vi "sendMessage.vi"(8 "error in (no error)":errorcluster, 10 "message":string, 11 "SpectrographClientCommunicator in":refnum<class "SpectrographClientCommunicator.lvclass">) -> (0 "error out":errorcluster, 3 "SpectrographClientCommunicator out":refnum<class "SpectrographClientCommunicator.lvclass">)   [LabVIEW 2016, in "SpectrographClientCommunicator.lvclass"]
uses:
  SpectrographClientCommunicator.lvclass
  ts_labview_tcp/TCPClient/TCPClient.lvclass
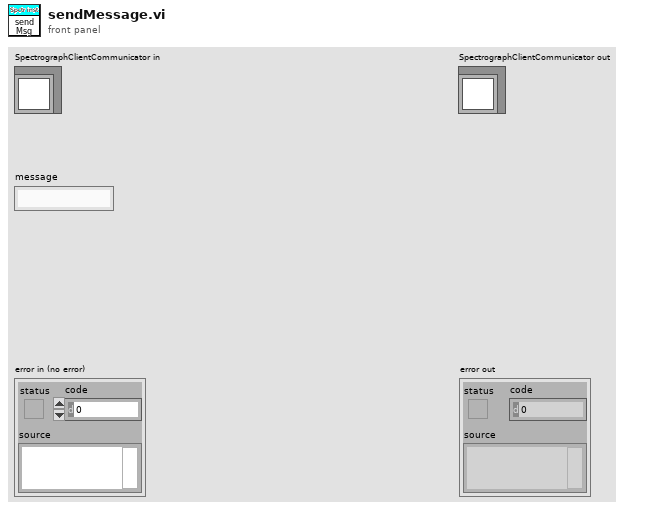
[diagram p1: front panel]
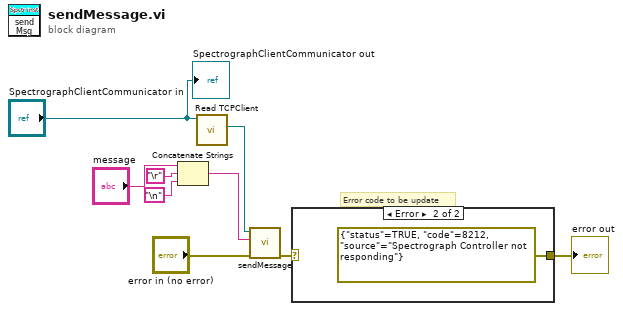
[diagram p0: block diagram]
diagram:
  # "Error code to be update"
  n1 = Concatenate Strings("message", "\r", "\n") -> (w6:string)
  n2 = call-dynamic "Read TCPClient.vi"("SpectrographClientCommunicator in"="SpectrographClientCommunicator in") -> ("TCPClient"=w4:refnum<class "TCPClient.lvclass">)  [unwired: 8 in, 2 out]
  n3 = call-dynamic "sendMessage.vi"("error in (no error)"="error in (no error)", "String"=w6, "TCPClient in"=w4) -> ("error out"=w2:errorcluster)  [unwired: 7 in, 1 out]
  n4 = case shown="Error" w2 {
    selector: w2 -> [w10 _]
    tunnel: [w10 errorcluster {"status"=TRUE, "code"=8212, "source"="Spectrograph Controller not responding"} ("error IO")] -> w1
    frame No Error {
    }
    frame Error {
    }
  }
  "error out" <- w1
  "SpectrographClientCommunicator out" <- "SpectrographClientCommunicator in"
